vi "Temperature Limit.vi"() -> ()   [LabVIEW 2015]
doc: "This VI simulates the acquisition of temperature, graphs the temperature, and notifies the user if the temperature is over the limit."
panel:
  in  "Start":bool
  in  "Delta t (ms)":i32(slide)=400 scale=50.0..500.0
  in  "Stop":bool
  in  "High Limit":dbl=28.0 format="%.2f"
  out "Temperature":cluster{"Temperature":dbl, "High Limit":dbl}(graph)={"Temperature"=85.88749999999999, "High Limit"=80.0}
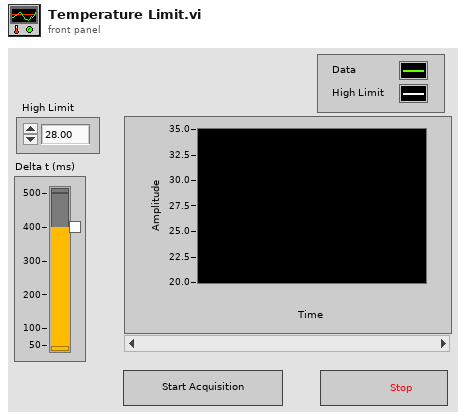
[diagram p1: front panel]
types:
  T1 = enum16{"Always On", "Always Off", "Off While Running"}
  T2 = cluster{"Temperature Value":dbl, "High Limit":dbl}
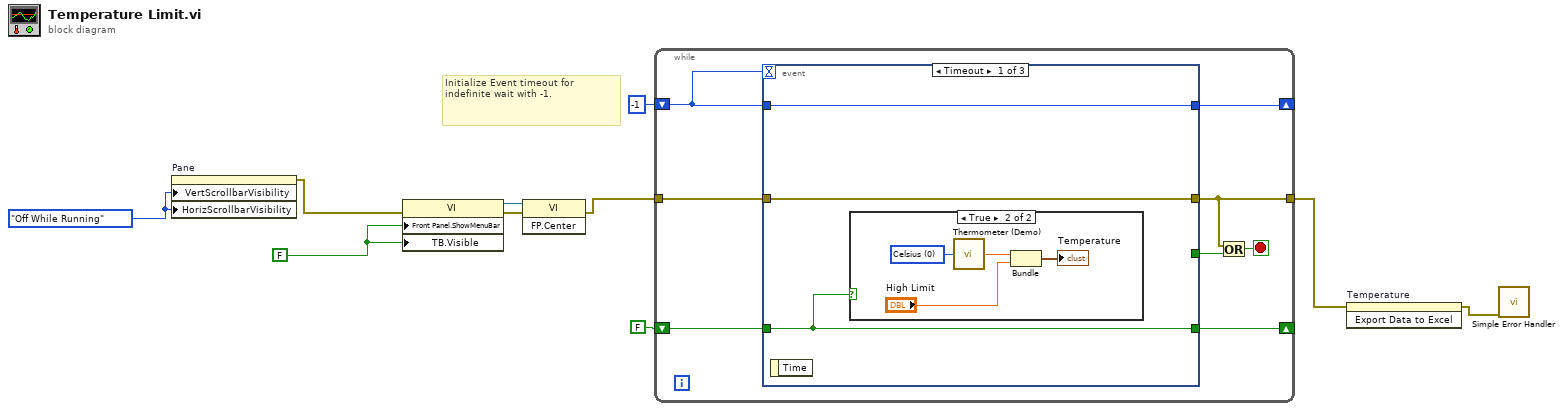
[diagram p0: block diagram]
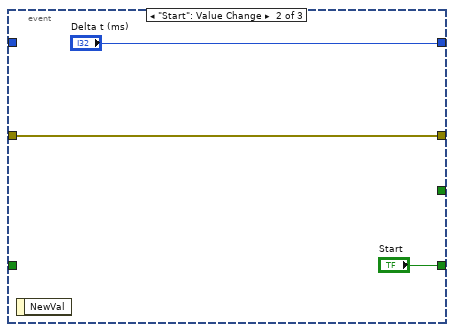
[diagram p3: hidden frame]
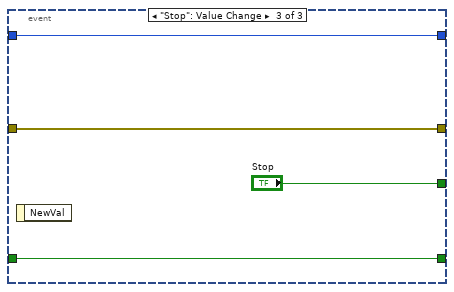
[diagram p4: hidden frame]
diagram:
  w7 = FALSE ("Front Panel Window:Show Menu Bar")
  w8 = T1."Off While Running" ("Vertical Scrollbar Visibility")
  # "Initialize Event timeout for indefinite wait with -1."
  n1 = property on="Pane" class="Pane"("VertScrollbarVisibility"=w8, "HorizScrollbarVisibility"=w8) -> (error out=w6:errorcluster)  [unwired: 2 in, 1 out]
  n2 = property class="VI"(error in=w6, "Front Panel.ShowMenuBar"=w7, "TB.Visible"=w7) -> (reference out=w5:refnum<vi>, error out=w4:errorcluster)  [unwired: 1 in]
  n3 = invoke class="VI" method="FP.Center"(reference=w5, error in=w4) -> (error out=w3:errorcluster)  [unwired: 1 in, 2 out]
  n4 = while {
    tunnel: w3 -> [w18]
    tunnel: [w16] -> w2
    shift-right: [w14] -> _
    shift-left: FALSE ("Start") -> [w13]
    shift-right: [w12] -> _
    shift-left: -1 ("Delta t (ms)") -> [w11]
    stop <- w17 stop-if-true
    n5 = event shown="[0] Timeout" {
      selector: _ -> [_ _ _]
      dyn-events: _ -> [_ _ _]
      timeout: w11 -> [_ _ _]
      tunnel: [_ _ "Stop"] -> w15
      tunnel: w18 -> [w21 w26 w31]
      tunnel: [w21 w26 w31] -> w16
      tunnel: [w19 "Start" w30] -> w14
      tunnel: w13 -> [w19 _ w30]
      tunnel: [w20 "Delta t (ms)" w29] -> w12
      tunnel: w11 -> [w20 _ w29]
      event Timeout {
        n6 = event-data() -> ()  [unwired: 1 in, 1 out]
        n7 = case shown="True" w19 {
          frame False {
          }
          frame True {
            w22 = u16 0 items=["Celsius", "Fahrenheit"] ("Units (0: Celsius)")
            n8 = call "Thermometer (Demo).vi"("Units (0: Celsius)"=w22) -> ("Temperature Value"=w23:dbl)
            n9 = Bundle("Temperature Value"=w23, "High Limit"="High Limit") -> (→"Temperature":T2)  [unwired: 1 in]
          }
        }
      }
      event "Start": Value Change {
        n10 = event-data() -> ()  [unwired: 1 in, 1 out]
      }
      event "Stop": Value Change {
        n11 = event-data() -> ()  [unwired: 1 in, 1 out]
      }
    }
    n12 = Or(x=w16, y=w15) -> (x .or. y?=w17:bool)
  }
  n13 = invoke on="Temperature" class="WFChart (strict)" method="Export Data to Excel"(error in=w2) -> (error out=w1:errorcluster)  [unwired: 2 in, 2 out]
  n14 = call <vilib>:"Simple Error Handler.vi"("error in (no error)"=w1) -> ()  [unwired: 4 in, 5 out]
